vi "Edit Plugin Type Specialization.vi"(11 "error in (no error)":errorcluster) -> (15 "error out":errorcluster)   [LabVIEW 2021, in "Migrator.lvlib"]
uses:
  Migrator.lvlib
  Path Functions/Path Functions.lvlib
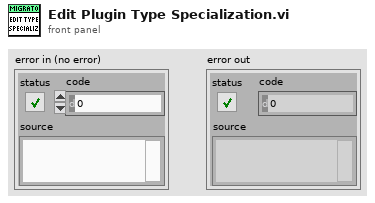
[diagram p1: front panel]
types:
  T1 = cluster{"parameter name":string, "type specialization":enum16{"none", "pin", "path", "enum"}, "annotations":cluster{"key":enum16{"none", "pin.instrument_type", "enum.values"}, "value":string}[]}[]
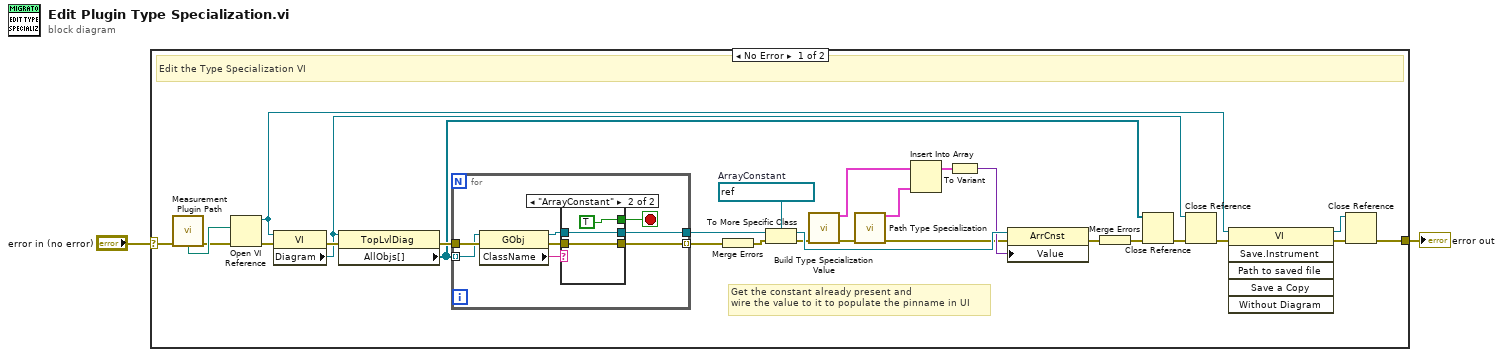
[diagram p0: block diagram]
diagram:
  n1 = case shown="No Error" "error in (no error)" {
    selector: "error in (no error)" -> [w7 w43]
    tunnel: [w22 w43] -> w1
    frame No Error {
      w20 = refnum<vi> refnum  # ArrayConstant
      # "Get the constant already present and\nwire the value to it to populate the pinname in UI"
      # "Edit the Type Specialization VI"
      n2 = call "Measurement Plugin Path.vi"("error in (no error)"=w7) -> ("Type Specialization"=w8:path, "error out"=w6:errorcluster)  [unwired: 2 in, 11 out]
      n3 = Open VI Reference(vi path=w8, error in (no error)=w6) -> (vi reference=w16:refnum<vi>, error out=w30:errorcluster)  [unwired: 4 in]
      n4 = property class="VI"(reference=w16, error in=w30) -> (error out=w29:errorcluster, "Diagram"=w23:refnum<vi>)  [unwired: 1 out]
      n5 = property class="TopLvlDiag"(reference=w23, error in=w29) -> (error out=w28:errorcluster, "AllObjs[]"=w24:refnum<vi>[])  [unwired: 1 out]
      n6 = for {
        tunnel: w24 -> [w37] mode=indexing
        tunnel: w28 -> [w38]
        tunnel: [w33] -> w21
        tunnel: [w31] -> w19 mode=indexing
        stop <- w32 stop-if-true
        n7 = property class="GObj"(reference=w37, error in=w38) -> (reference out=w34:refnum<vi>, error out=w35:errorcluster, "ClassName"=w36:string)
        n8 = case shown="\"ArrayConstant\"" w36 {
          tunnel: w35 -> [w39 w40]
          tunnel: w34 -> [_ w42]
          tunnel: [_ w42] -> w33
          tunnel: [_ TRUE] -> w32
          tunnel: [w39 w40] -> w31
          frame Default {
          }
          frame "ArrayConstant" {
          }
        }
      }
      n9 = Merge Errors(w19) -> (w18:errorcluster)
      n10 = To More Specific Class(target class=w20, reference=w21, error in=w18) -> (specific class reference=w15:refnum<vi>, error out=w14:errorcluster)
      n11 = call "Build Type Specialization Value.vi"("error in (no error)"=w14) -> ("Type Specialization"=w10:T1, "error out"=w4:errorcluster)  [unwired: 13 in]
      n12 = call "Path Type Specialization.vi"("error in (no error)"=w4) -> ("Type Specialization for Path"=w5:T1, "error out"=w3:errorcluster)  [unwired: 13 in]
      n13 = Insert Into Array(array=w10, new element=w5) -> (w9:T1)  [unwired: 1 in]
      n14 = To Variant(anything=w9) -> (Variant=w13:variant)
      n15 = property class="ArrCnst"(reference=w15, error in=w3, "Value"=w13) -> (error out=w12:errorcluster)  [unwired: 1 out]
      n16 = Merge Errors(w12) -> (w27:errorcluster)
      n17 = Close Reference(reference=w24, error in (no error)=w27) -> (error out=w26:errorcluster)
      n18 = Close Reference(reference=w23, error in (no error)=w26) -> (error out=w25:errorcluster)
      n19 = invoke class="VI" method="Save.Instrument"(reference=w16, error in=w25) -> (reference out=w11:refnum<vi>, error out=w17:errorcluster)  [unwired: 4 in, 4 out]
      n20 = Close Reference(reference=w11, error in (no error)=w17) -> (error out=w22:errorcluster)
    }
    frame Error {
    }
  }
  "error out" <- w1
